vi "Share external clock.vi"() -> ()   [LabVIEW 2012]
uses:
  <vilib>/Platform/TimedLoop/XDataNode/timing_clust.ctl
  <vilib>/Platform/TimedLoop/XDataNode/nitl_modes.ctl
  <vilib>/Platform/TimedLoop/XDataNode/wakeup.ctl
  <vilib>/rvi/Emulation/niFpgaSctlEmulationRegisterWithScheduler.vi
  <vilib>/rvi/Emulation/niFpgaSctlEmulationScheduler.vi
  <vilib>/rvi/eio/common/nirviEmuTemplateMethod_errors.vi
  <vilib>/Platform/TimedLoop/XDataNode/XDataNode.xnode
  <vilib>/eio/EIONode/EIONode.xnode
  <vilib>/Platform/TimedLoop/XDataNode/XDNodeRunTimeDep.lvlib
panel:
  out "Falling Edge Trigger LED":bool
  out "Rising Edge Trigger LED":bool
  out "Clock":bool
  in  "stop":bool
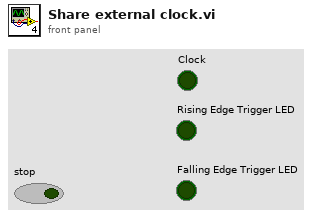
[diagram p1: front panel]
types:
  T1 = typedef "XDNodeRunTimeDep.lvlib/timing_clust.ctl" = cluster{"Expected End [f-1]":u64, "Actual End [f-1]":u64, "Finished Late? [f-1]":bool, "Expected End [i-1]":u64, "Actual End [i-1]":u64, "Finished Late? [i-1]":bool, "Expected Start [i]":u64, "Actual Start [i]":u64, "Expected Start [f]":u64, "Actual Start [f]":u64, "Source Name":string, "Structure Name":string, "Period":i64, "Deadline":i64, "Offset":i64, "Start":i64, "Priority":i32, "Timeout":i32, "Mode":T2, "Wakeup Reason":T3, "Error":errorcluster, "Source Type":string, "Secondary Source Type":string, "Global End Time":u64, "Global Start Time":u64, "Frame Duration":u64, "Iteration Duration":u64, "Assigned CPU":i32, "I/O Scan Engine Mode":u32}
  T2 = typedef "XDNodeRunTimeDep.lvlib/nitl_modes.ctl" = enum32{"No Change", "Process missed periods, maintain original phase", "Discard missed periods, maintain original phase", "Process missed periods, ignore original phase", "Discard missed periods, ignore original phase"}
  T3 = typedef "XDNodeRunTimeDep.lvlib/wakeup.ctl" = enum32{"Normal", "Aborted", "Asynchronous wakeup", "Timing source error", "Timed loop error", "Timeout"}
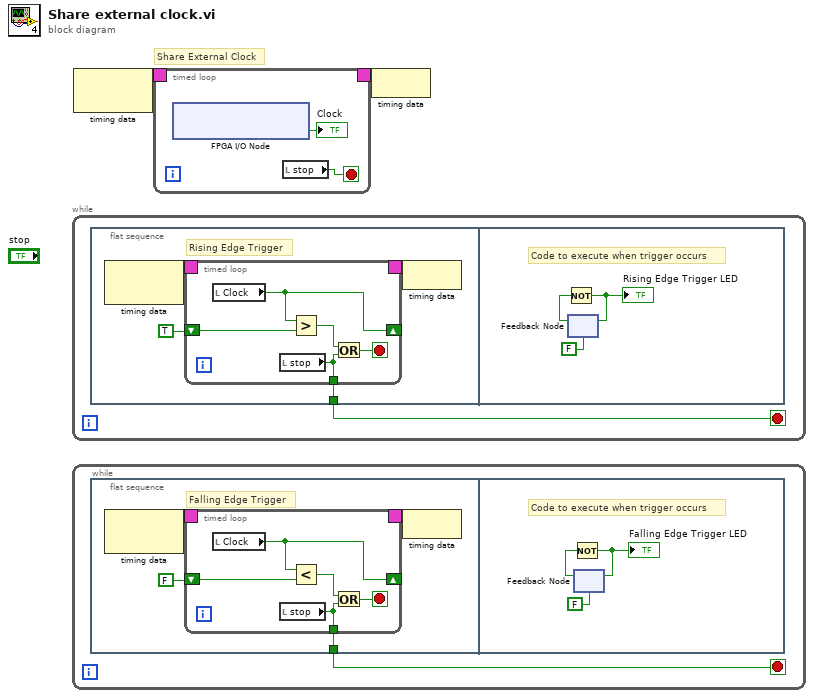
[diagram p0: block diagram]
diagram:
  # "Share External Clock"
  n1 = while {
    stop <- w3 stop-if-true
    n2 = flat-sequence {
      tunnel: [w4] -> w3
      frame #0 {
        # "Rising Edge Trigger"
        n3 = node-c288 ("Rising Edge Trigger")() -> (w7:T1)  [unwired: 1 in]
        n4 = timed-loop "Rising Edge Trigger" {
          timing: w7 -> [_]
          timing-out: [_] -> w6
          shift-right: [w11] -> _
          shift-left: TRUE -> [w12]
          tunnel: [w8] -> w4
          stop <- w9 stop-if-true
          n5 = local read "Clock"() -> (w11:bool)
          n6 = local read "stop"() -> (w8:bool)
          n7 = Greater?(x=w11, y=w12) -> (0:w10:bool)
          n8 = Or(x=w10, y=w8) -> (x .or. y?=w9:bool)
        }
        n9 = node-c288(w6) -> ()
      }
      frame #1 {
        # "Code to execute when trigger occurs"
        n10 = feedback #1(FALSE) -> (w17:bool)
        n11 = Not(x=w17) -> (.not. x?=w18:bool)
        "Rising Edge Trigger LED" <- w18
        n12 = feedback-in #1(w18) -> ()
      }
    }
  }
  n13 = while {
    stop <- w20 stop-if-true
    n14 = flat-sequence {
      tunnel: [w21] -> w20
      frame #0 {
        # "Falling Edge Trigger"
        n15 = node-c288 ("Rising Edge Trigger")() -> (w24:T1)  [unwired: 1 in]
        n16 = timed-loop "Falling Edge Trigger" {
          timing: w24 -> [_]
          timing-out: [_] -> w23
          shift-right: [w28] -> _
          shift-left: FALSE -> [w29]
          tunnel: [w25] -> w21
          stop <- w26 stop-if-true
          n17 = local read "Clock"() -> (w28:bool)
          n18 = local read "stop"() -> (w25:bool)
          n19 = Less?(x=w28, y=w29) -> (x < y?=w27:bool)
          n20 = Or(x=w27, y=w25) -> (x .or. y?=w26:bool)
        }
        n21 = node-c288(w23) -> ()
      }
      frame #1 {
        # "Code to execute when trigger occurs"
        n22 = feedback #2(FALSE) -> (w36:bool)
        n23 = Not(x=w36) -> (.not. x?=w35:bool)
        "Falling Edge Trigger LED" <- w35
        n24 = feedback-in #2(w35) -> ()
      }
    }
  }
  n25 = node-c288() -> (w2:T1)  [unwired: 1 in]
  n26 = timed-loop "Share External Clock" {
    timing: w2 -> [_]
    timing-out: [_] -> w1
    stop <- w37 stop-if-true
    n27 = xnode "FPGA I/O Node"() -> ("Connector0/DIO0"=→"Clock":bool)  [unwired: 1 in, 1 out]
    n28 = local read "stop"() -> (w37:bool)
  }
  n29 = node-c288(w1) -> ()
